vi "Excel Easy Text.vi"(0 "report in":refnum<class "NI_report.lvclass">, 1 "border? (F)":bool, 2 "font":T1={"font name"="", "font size"=10.0, "bold"=0, "italic"=0, "underline"=0, "strike through"=0, "font color"=16777216} {"font size" format="%0.2f"; "strike through" items=["Unchanged", "Yes", "No"]; "underline" items=["Unchanged", "Yes", "No"]; "italic" items=["Unchanged", "Yes", "No"]; "bold" items=["Unchanged", "Yes", "No"]}, 3 "font settings source":u16(ring) items=["VI Inputs", "Font Dialog Box"], 5 "text":string, 7 "start (-1, -1)":cluster{"row":i32, "column":i32}={"row"=-1, "column"=-1}, 9 "end (-1, -1)":cluster{"row":i32, "column":i32}={"row"=-1, "column"=-1}, 11 "error in (no error)":errorcluster, 12 "name (\"\")":string) -> (4 "report out":refnum<class "NI_report.lvclass">, 6 "font out":T1={"font name"="", "font size"=10.0, "bold"=0, "italic"=0, "underline"=0, "strike through"=0, "font color"=16777216} {"font size" format="%0.2f"; "strike through" items=["Unchanged", "Yes", "No"]; "underline" items=["Unchanged", "Yes", "No"]; "italic" items=["Unchanged", "Yes", "No"]; "bold" items=["Unchanged", "Yes", "No"]}, 8 "next cell bottom-left":cluster{"row":i32, "column":i32}, 10 "next cell top-right":cluster{"row":i32, "column":i32}, 15 "error out":errorcluster)   [LabVIEW 2010, in "NI_ReportGenerationToolkit.lvlib"]
doc: "Inserts text into a Microsoft Excel report."
uses:
  <vilib>/addons/_office/NI_ReportGenerationToolkit.lvlib
  <vilib>/Utility/NIReport.llb/NI_report.lvclass
  <vilib>/addons/_office/_exclsub.llb/font.ctl
  <vilib>/Utility/NIReport.llb/Excel/NI_Excel.lvclass
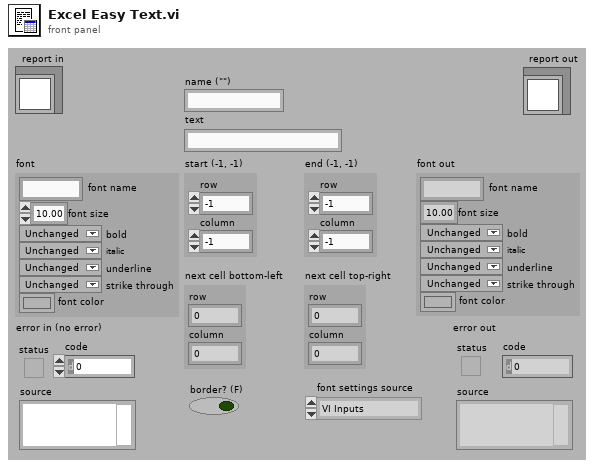
[diagram p1: front panel]
types:
  T1 = typedef "NI_ReportGenerationToolkit.lvlib/font.ctl" = cluster{"font name":string, "font size":dbl, "bold":u16, "italic":u16, "underline":u16, "strike through":u16, "font color":u32}
  T2 = cluster{"on/off":bool, "weight":i32, "color":u32}
  T3 = cluster{"Charset (-1)":i16, "Weight (-1)":i16, "Name":string, "Size":string}
  T4 = cluster{"position (Excel)":cluster{"row":i32, "column":i32}, "name (Excel)":string, "bookmark (Word)":string}
  T5 = cluster{"italic":u16, "strike through":u16, "underline":u16, "bold":u16}
  T6 = cluster{i32, i32, i32, i32, "charset":i16, "weight":i16, "name":string, "size":string, "text color":u32}
  T7 = typedef "NI_ReportGenerationCore.lvlib/font.ctl" = cluster{"font name":string, "font size":dbl, "bold":u16, "italic":u16, "underline":u16, "strike through":u16, "font color":u32}
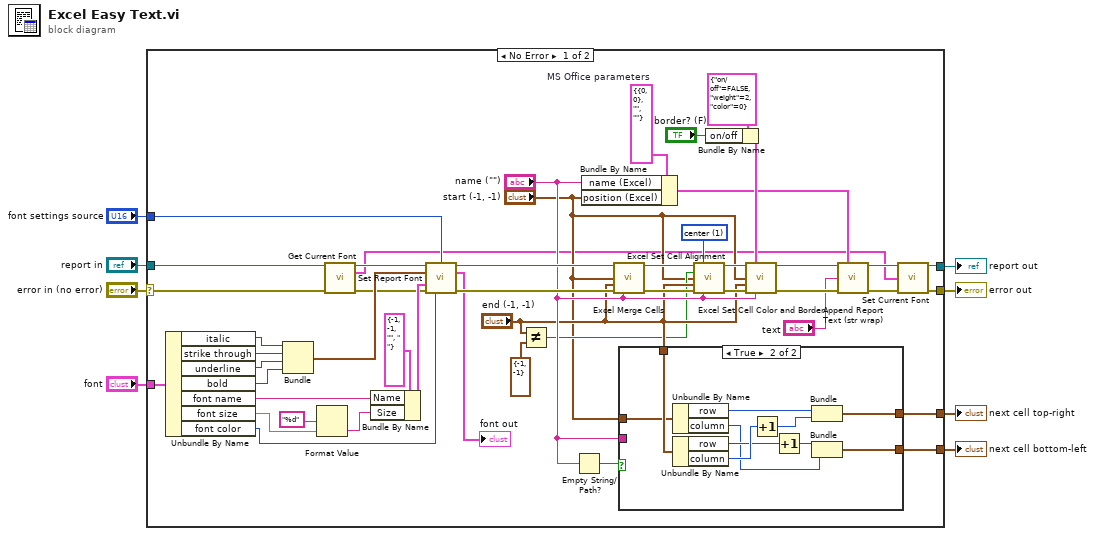
[diagram p0: block diagram]
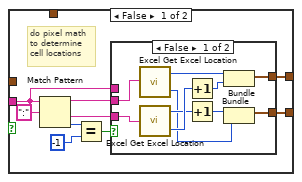
[diagram p2: hidden frame]
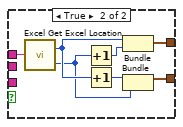
[diagram p3: hidden frame]
diagram:
  n1 = case shown="No Error" "error in (no error)" {
    selector: "error in (no error)" -> [w19 w92]
    tunnel: "font" -> [w37 _]
    tunnel: [w36 _] -> w7
    tunnel: [w35 _] -> w6
    tunnel: "report in" -> [w22 w93]
    tunnel: [w10 w92] -> w4
    tunnel: [w11 w93] -> w3
    tunnel: "font settings source" -> [w21 _]
    frame No Error {
      w53 = T4 {"position (Excel)"={"row"=0, "column"=0}, "name (Excel)"="", "bookmark (Word)"=""}  # MS Office parameters
      w30 = 1 items=["top", "center", "bottom"] ("vertical alignment")
      n2 = Unbundle By Name(w37) -> ("italic"=w42:u16, "strike through"=w45:u16, "underline"=w44:u16, "bold"=w43:u16, "font name"=w41:string, "font size"=w47:dbl, "font color"=w38:u32)
      n3 = Bundle("italic"=w42, "strike through"=w45, "underline"=w44, "bold"=w43) -> (w39:T5)  [unwired: 1 out]
      n4 = Format Value(format string="%d", value (0)=w47) -> (output string=w40:string)  [unwired: 1 out]
      n5 = call <vilib>:"Get Current Font.vi"("report in"=w22, "error in (no error)"=w19) -> ("report.lvclass"=w23:refnum<class "NI_report.lvclass">, "font"=w9:T6, "error out"=w24:errorcluster)  [unwired: 11 out]
      n6 = Bundle By Name(cluster=T3 {"Charset (-1)"=-1, "Weight (-1)"=-1, "Name"="", "Size"=" "} ("font settings"), "Name"=w41, "Size"=w40) -> (w55:T3)
      n7 = call-dynamic "Set Report Font.vi"("report in"=w23, "text color (unchanged)"=w38, "font settings source"=w21, "text options"=w39, "font settings"=w55, "error in (no error)"=w24) -> ("report out"=w52:refnum<class "NI_report.lvclass">, "font out"=→"font out":T7, "error out"=w51:errorcluster)  [unwired: 7 in]
      n8 = Not Equal?(x="end (-1, -1)", y=cluster{"row":i32, "column":i32} {"row"=-1, "column"=-1}) -> (x != y?=w25:bool)
      n9 = Empty String/Path?(string/path="name (\"\")") -> (empty?=w29:bool)
      n10 = Bundle By Name(cluster=w53, "name (Excel)"="name (\"\")", "position (Excel)"="start (-1, -1)") -> (w14:T4)
      n11 = call <vilib>:"Excel Merge Cells.vi"("report in"=w52, "start (-1, -1)"="start (-1, -1)", "end (-1, -1)"="end (-1, -1)", "error in (no error)"=w51, "name (\"\")"="name (\"\")") -> ("report out"=w33:refnum<class "NI_report.lvclass">, "error out"=w34:errorcluster)  [unwired: 9 out]
      n12 = case shown="True" w29 {
        tunnel: "end (-1, -1)" -> [_ w85]
        tunnel: [w59 w84] -> w36
        tunnel: [w58 w83] -> w35
        tunnel: "start (-1, -1)" -> [_ w82]
        tunnel: "name (\"\")" -> [w60 _]
        frame False {
          # "do pixel math\nto determine\ncell locations"
          n13 = Match Pattern(string=w60, regular expression=":") -> (before substring=w57:string, after substring=w56:string, offset past match=w63:i32)  [unwired: 2 out]
          n14 = Equal?(x=w63, y=-1) -> (x = y?=w61:bool)
          n15 = case shown="False" w61 {
            tunnel: w60 -> [_ w81]
            tunnel: [w69 w79] -> w59
            tunnel: [w65 w75] -> w58
            tunnel: w57 -> [w74 _]
            tunnel: w56 -> [w73 _]
            frame False {
              n16 = call <vilib>:"Excel Get Excel Location.vi"("cell's name"=w74) -> ("row"=w72:i32, "column"=w66:i32)
              n17 = call <vilib>:"Excel Get Excel Location.vi"("cell's name"=w73) -> ("row"=w68:i32, "column"=w71:i32)
              n18 = Increment(x=w71) -> (x+1=w70:i32)
              n19 = Increment(x=w68) -> (x+1=w67:i32)
              n20 = Bundle("row"=w72, w70) -> (w69:cluster{"row":i32, i32})  [unwired: 1 out]
              n21 = Bundle(w67, "column"=w66) -> (w65:cluster{i32, "column":i32})  [unwired: 1 out]
            }
            frame True {
              n22 = call <vilib>:"Excel Get Excel Location.vi"("cell's name"=w81) -> ("row"=w78:i32, "column"=w77:i32)
              n23 = Increment(x=w77) -> (x+1=w80:i32)
              n24 = Increment(x=w78) -> (x+1=w76:i32)
              n25 = Bundle("row"=w78, w80) -> (w79:cluster{"row":i32, i32})  [unwired: 1 out]
              n26 = Bundle(w76, "column"=w77) -> (w75:cluster{i32, "column":i32})  [unwired: 1 out]
            }
          }
        }
        frame True {
          n27 = Unbundle By Name(w82) -> ("row"=w91:i32, "column"=w86:i32)
          n28 = Unbundle By Name(w85) -> ("row"=w88:i32, "column"=w90:i32)
          n29 = Increment(x=w90) -> (x+1=w89:i32)
          n30 = Increment(x=w88) -> (x+1=w87:i32)
          n31 = Bundle("row"=w91, w89) -> (w84:cluster{"row":i32, i32})  [unwired: 1 out]
          n32 = Bundle(w87, "column"=w86) -> (w83:cluster{i32, "column":i32})  [unwired: 1 out]
        }
      }
      n33 = call <vilib>:"Excel Set Cell Alignment.vi"("report in"=w33, "vertical alignment (top)"=w30, "wrap text? (F)"=w25, "start (-1, -1)"="start (-1, -1)", "end (-1, -1)"="end (-1, -1)", "error in (no error)"=w34, "name (\"\")"="name (\"\")") -> ("report out"=w31:refnum<class "NI_report.lvclass">, "error out"=w32:errorcluster)  [unwired: 1 in, 6 out]
      n34 = Bundle By Name(cluster=T2 {"on/off"=FALSE, "weight"=2, "color"=0} ("inside border"), "on/off"="border? (F)") -> (w49:T2)
      n35 = call <vilib>:"Excel Set Cell Color and Border.vi"("report in"=w31, "inside border"=w49, "start (-1, -1)"="start (-1, -1)", "end (-1, -1)"="end (-1, -1)", "error in (no error)"=w32, "name (\"\")"="name (\"\")") -> ("report out"=w17:refnum<class "NI_report.lvclass">, "error out"=w16:errorcluster)  [unwired: 2 in, 6 out]
      n36 = call <vilib>:"Append Report Text (str wrap).vi"("report in"=w17, "MS Office parameters"=w14, "text"="text", "error in (no error)"=w16) -> ("report out"=w12:refnum<class "NI_report.lvclass">, "error out"=w13:errorcluster)  [unwired: 2 in, 8 out]
      n37 = call <vilib>:"Set Current Font.vi"("report in"=w12, "font"=w9, "error in (no error)"=w13) -> ("report out"=w11:refnum<class "NI_report.lvclass">, "error out"=w10:errorcluster)  [unwired: 11 out]
    }
    frame Error {
    }
  }
  "report out" <- w3
  "error out" <- w4
  "next cell bottom-left" <- w6
  "next cell top-right" <- w7
